vi "Sub_Python_node_eigh.vi"(10 "Stiff":T1, 11 "Mass":T1) -> (2 "Eigenvectors":T1, 3 "Eigenvals":T1)   [LabVIEW 2019]
uses:
  <vilib>/Analysis/Matrix/Datatypes/RealMatrix.ctl
  <vilib>/Analysis/Matrix/Numeric/Conversions/Array To Matrix - RA2.vi
  <vilib>/Analysis/Matrix/NI_Matrix.lvlib
panel:
  # "The Bitedness of LabView is 32 and the Bitedness of the python installation is 64 this will not work without uninstalling Anaconda and reinstalling it as 32bit see getEigenCommandPrompt.vi prompt for the work around"
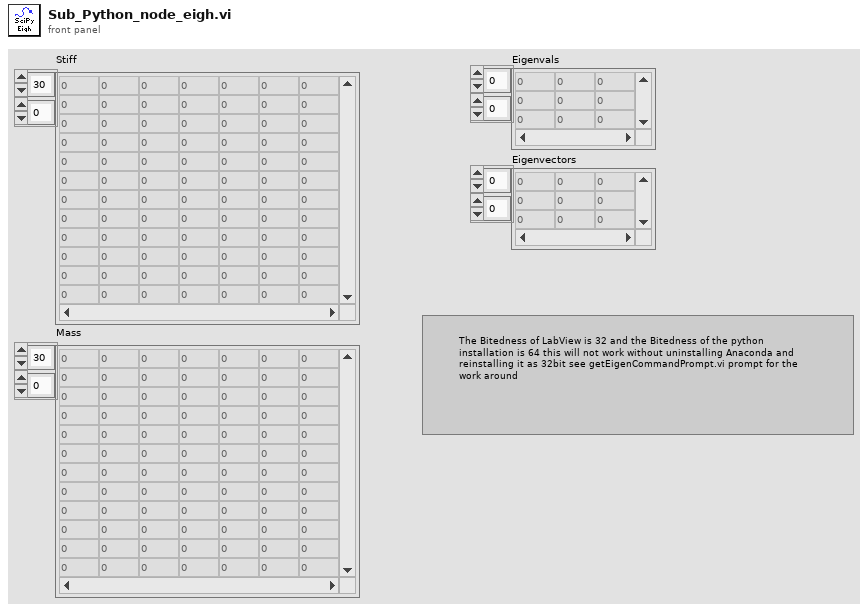
[diagram p1: front panel]
types:
  T1 = typedef "NI_Matrix.lvlib/RealMatrix.ctl" = dbl[][]
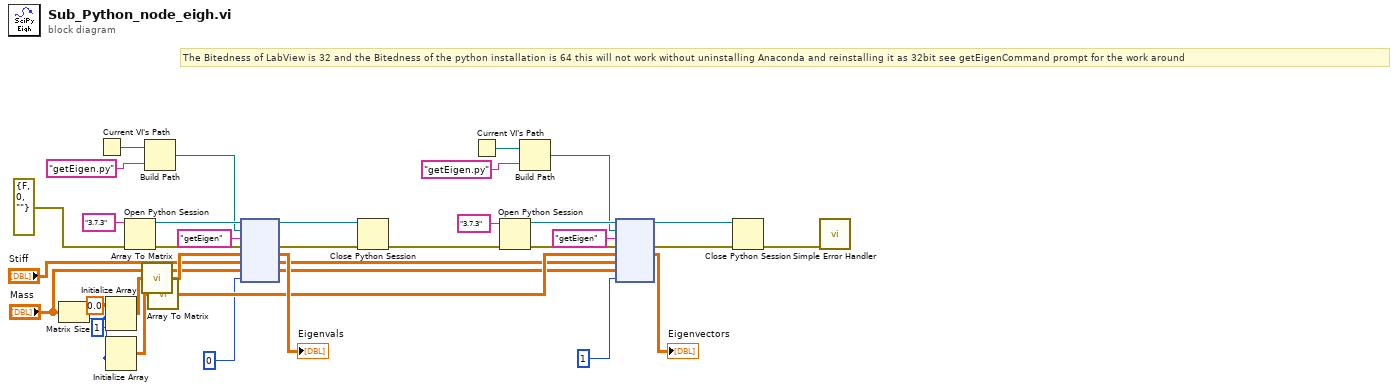
[diagram p0: block diagram]
diagram:
  w27 = 0.0 ("element")
  # "The Bitedness of LabView is 32 and the Bitedness of the python installation is 64 this will not work without uninstalling Anaconda and reinstalling it as 32bit see getEigenCommand prompt for the work around"
  n1 = Matrix Size(0:"Mass") -> (2:w28:i32)  [unwired: 1 out]
  n2 = Current VI's Path() -> (path=w23:path)
  n3 = Initialize Array(w27, w28, 1 ("dimension size")) -> (w29:dbl[][])
  n4 = Initialize Array(w27, w28, w28) -> (w26:dbl[][])
  n5 = Open Python Session(python version="3.7.3" ("Python version"), 3:errorcluster {"status"=FALSE, "code"=0, "source"=""} ("error in (no error)")) -> (session out=w32:refnum<k35>, error out=w21:errorcluster)  [unwired: 1 in]
  n6 = call-poly <vilib>:"Array To Matrix.vi"("Real 2D Array"=w29) -> ("Real Matrix"=w8:T1)
  n7 = Build Path(base path=w23, name or relative path="getEigen.py" ("function name")) -> (appended path=w20:path)
  n8 = call-poly <vilib>:"Array To Matrix.vi"("Real 2D Array"=w26) -> ("Real Matrix"=w6:T1)
  n9 = node ("Python Node")(w32, w20, "getEigen" ("function name"), w21, w8, "Stiff", "Mass", 0) -> (w31:refnum<k35>, w33:errorcluster, →"Eigenvals":T1)  [unwired: 3 in, 2 out]
  n10 = Close Python Session(session in=w31, error in=w33) -> (11:w9:errorcluster)
  n11 = Current VI's Path() -> (path=w13:path)
  n12 = Open Python Session(python version="3.7.3" ("Python version"), 3:w9) -> (session out=w18:refnum<k35>, error out=w11:errorcluster)  [unwired: 1 in]
  n13 = Build Path(base path=w13, name or relative path="getEigen.py" ("function name")) -> (appended path=w10:path)
  n14 = node ("Python Node")(w18, w10, "getEigen" ("function name"), w11, w6, "Stiff", "Mass", 1) -> (w17:refnum<k35>, w19:errorcluster, →"Eigenvectors":T1)  [unwired: 3 in, 2 out]
  n15 = Close Python Session(session in=w17, error in=w19) -> (11:w14:errorcluster)
  n16 = call <vilib>:"Simple Error Handler.vi"("error in (no error)"=w14) -> ()  [unwired: 4 in, 5 out]
